vi "helper- line ROI to 2 UTM Pts.vi"(2 "ROI":T2, 3 "Image Descriptor":T3={"Upper-Left Corner Coordinates"={"UTM Zone"=0.0, "Hemisphere"=enum."North", "East"=0.0, "North"=0.0}, "Meters/Pixel"=42.294203} {"Upper-Left Corner Coordinates"."North" format="%#_10f"; "Upper-Left Corner Coordinates"."East" format="%#_8f"}) -> (0 "Endpoint UTM 2":T1 {"North" format="%#_10f"; "East" format="%#_8f"}, 1 "Endpoint UTM 1":T1 {"North" format="%#_10f"; "East" format="%#_8f"})   [LabVIEW 2011]
doc: "takes in an ROI such as that produced by the line tool, along with an image descriptor, and outputs the UTM locations of the line's endpoints."
uses:
  mission input/0-Image Descriptor.ctl
  2-Think/2 Typedefs/UTM Location.ctl
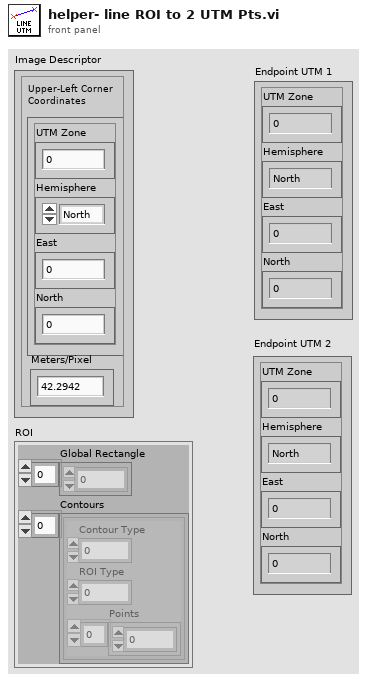
[diagram p1: front panel]
types:
  T1 = typedef "UTM Location.ctl" = cluster{"UTM Zone":dbl, "Hemisphere":enum16{"North", "South"}, "East":dbl, "North":dbl}
  T2 = cluster{"Global Rectangle":i32[], "Contours":cluster{"Contour Type":u32, "ROI Type":u32, "Points":i32[]}[]}
  T3 = typedef "0-Image Descriptor.ctl" = cluster{"Upper-Left Corner Coordinates":T1, "Meters/Pixel":dbl}
  T4 = cluster{"Contour Type":u32, "ROI Type":u32, "Points":i32[]}[]
  T5 = cluster{"Contour Type":u32, "ROI Type":u32, "Points":i32[]}
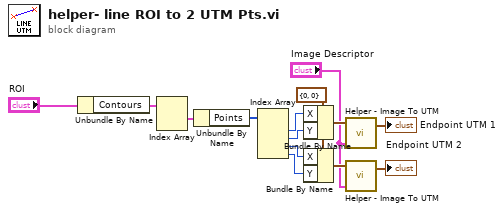
[diagram p0: block diagram]
diagram:
  w9 = cluster{"X":i32, "Y":i32} {"X"=0, "Y"=0} ("Pixel Coordinates")
  n1 = Unbundle By Name("ROI") -> ("Contours"=w14:T4)
  n2 = Index Array(array=w14) -> (element #1=w13:T5)  [unwired: 2 in, 1 out]
  n3 = Unbundle By Name(w13) -> ("Points"=w11:i32[])
  n4 = Index Array(array=w11) -> (element #1=w8:i32, element #2=w7:i32, element #3=w6:i32, element #4=w5:i32)  [unwired: 4 in]
  n5 = Bundle By Name(cluster=w9, "X"=w8, "Y"=w7) -> (w12:cluster{"X":i32, "Y":i32})
  n6 = Bundle By Name(cluster=w9, "X"=w6, "Y"=w5) -> (w10:cluster{"X":i32, "Y":i32})
  n7 = call "Helper - Image To UTM.vi"("Image Descriptor"="Image Descriptor", "Pixel Coordinates"=w12) -> ("UTM Location"=→"Endpoint UTM 1":T1)  [unwired: 1 in, 1 out]
  n8 = call "Helper - Image To UTM.vi"("Image Descriptor"="Image Descriptor", "Pixel Coordinates"=w10) -> ("UTM Location"=→"Endpoint UTM 2":T1)  [unwired: 1 in, 1 out]
